vi "INI.Attributes to Variant.vi"(8 "error in (no error)":errorcluster, 9 "Section Attribute":variant, 10 "Data Name":string, 11 "Datatype":variant) -> (0 "error out":errorcluster, 3 "Variant":variant)   [LabVIEW 2013, in "OpenSerializer.lvlib" / "Serializer.PlainText.INI.lvclass"]
doc: "JKI SMO Configuration 1.2.1.18\nJKI - JKI\nCopyright (c) 2017, JKI"
uses:
  Serializer.PlainText.INI.lvclass
  <vilib>/LabVIEW Open Source Project/Data Manipulation/TypeDescriptor/TypeDescriptor_GetName.vi
  <vilib>/LabVIEW Open Source Project/Data Manipulation/Variant/Variant_EmptyCluster.vi
  <vilib>/LabVIEW Open Source Project/Data Manipulation/TypeDescriptor/TypeDescriptor_GetPString.vi
  <vilib>/LabVIEW Open Source Project/Data Manipulation/TypeDescriptor/TypeDescriptor_SetName.vi
  <vilib>/Utility/GetType.llb/TD_Create Cluster.vi
  <vilib>/Utility/GetType.llb/TD_Get Array Information.vi
  <vilib>/Utility/GetType.llb/Get Type Code from I16 Array And Pos.vi
  <vilib>/LabVIEW Open Source Project/Data Manipulation/Conversions/Flattened nD-Array to Flattened 1D-Array.vi
  <vilib>/regexp/Match Regular Expression.xnode
  <vilib>/Utility/VariantDataType/VariantType.lvlib
  <vilib>/LabVIEW Open Source Project/Data Manipulation/Variant/OpenVariant.lvlib
  Serializer.PlainText/Serializer.PlainText.lvclass
  <vilib>/LabVIEW Open Source Project/Data Manipulation/TypeDescriptor/OpenDescriptor.lvlib
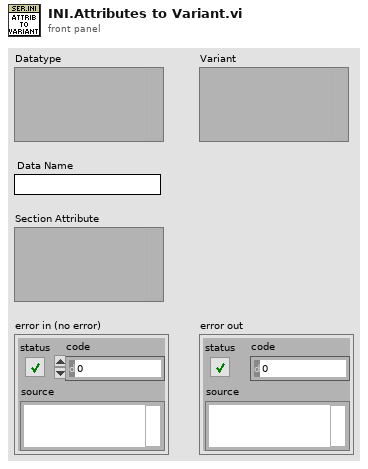
[diagram p1: front panel]
types:
  T1 = typedef "VariantType.lvlib/Type.ctl" = enum8{"Invalid Type", "Void", "I8", "I16", "I32", "I64", "U8", "U16", "U32", "U64", "Single Float", "Double Float", "Extended Float", "Single Complex", "Double Complex", "Extended Complex", "Enum U8", "Enum U16", "Enum U32", "Enum U64", "Single Float With Unit", "Double Float With Unit", "Extended Float With Unit", "Single Complex with Unit", "Double Complex with Unit", "Extended Complex with Unit", "Boolean", "String", "Path", "Picture", "Tag", "Array", "Cluster", "Variant", "LV Variant", "Waveform", "Timestamp", "Digital Waveform", "Digital Data", "ExpressData", "Refnum", "External Data", "VI", "Poly VI", "LabVIEW Class Instance", "Fixed Point"}
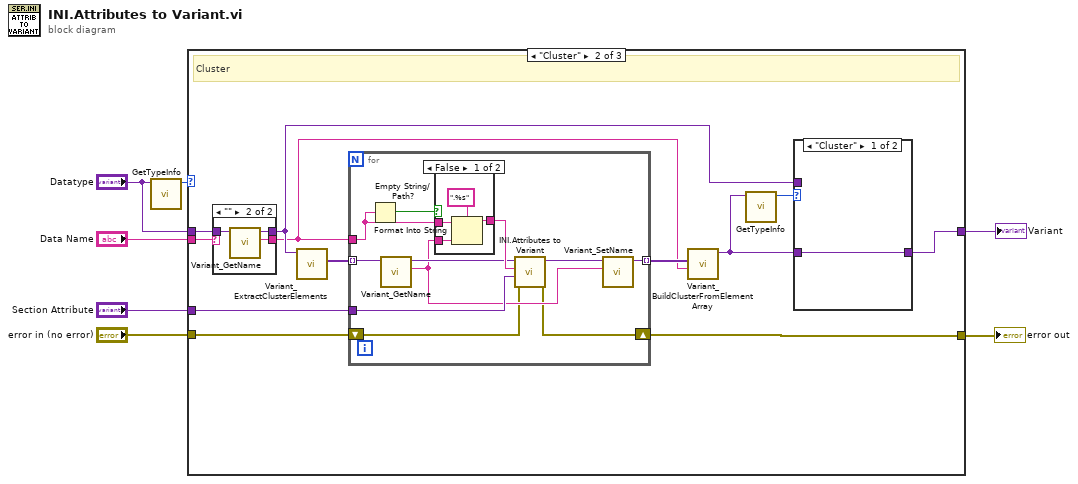
[diagram p0: block diagram]
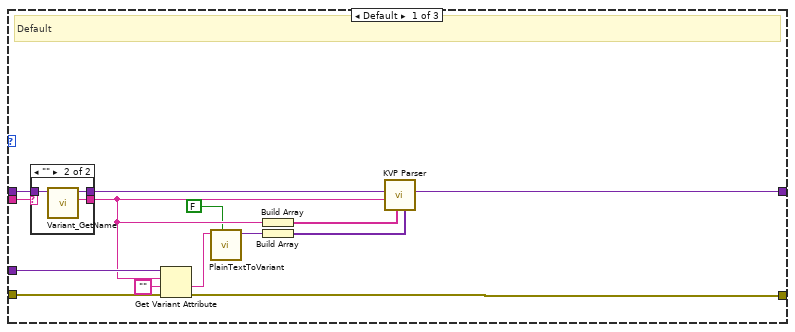
[diagram p2: hidden frame]
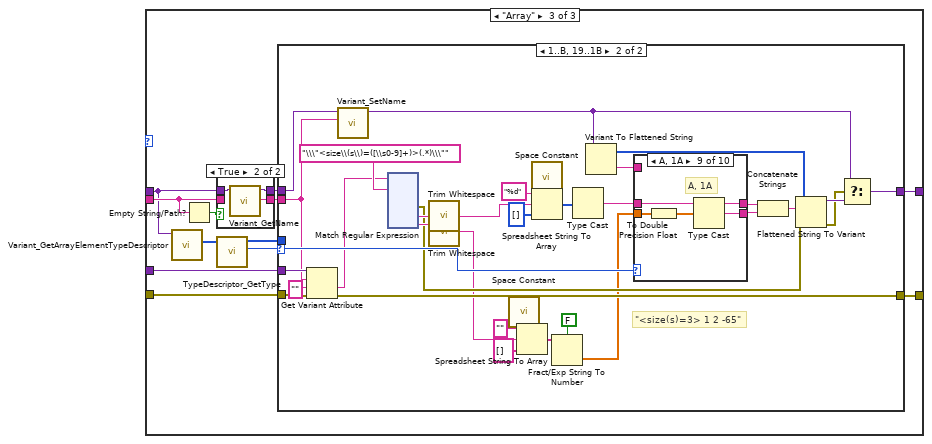
[diagram p7: hidden frame]
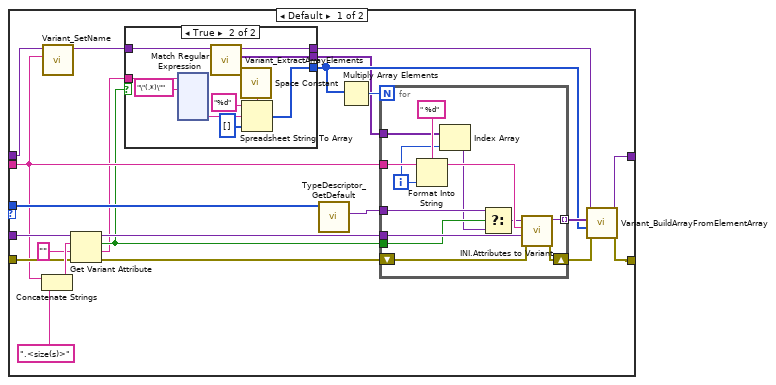
[diagram p9: hidden frame]
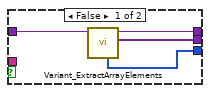
[diagram p10: hidden frame]
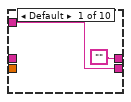
[diagram p11: hidden frame]
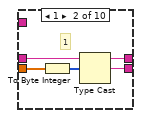
[diagram p12: hidden frame]
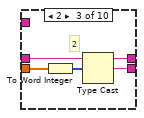
[diagram p13: hidden frame]
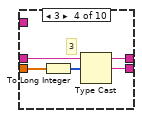
[diagram p14: hidden frame]
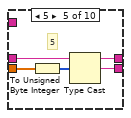
[diagram p15: hidden frame]
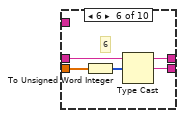
[diagram p16: hidden frame]
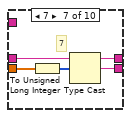
[diagram p17: hidden frame]
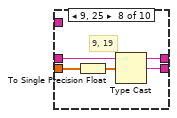
[diagram p18: hidden frame]
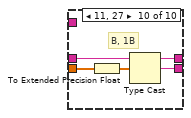
[diagram p19: hidden frame]
diagram:
  n1 = call <vilib>:"GetTypeInfo.vi"("Variant"="Datatype") -> ("Type Enum"=w1:T1)  [unwired: 6 in, 4 out]
  n2 = case shown="\"Cluster\"" w1 {
    tunnel: [w9 w37 w72] -> w3
    tunnel: [w20 w33 w71] -> w4
    tunnel: "Data Name" -> [w18 w27 w67]
    tunnel: "Datatype" -> [w19 w30 w65]
    tunnel: "Section Attribute" -> [w21 w38 w73]
    tunnel: "error in (no error)" -> [w12 w31 w66]
    frame Default {
      # "Default"
      n3 = case shown="\"\"" w18 {
        selector: w18 -> [w22 _]
        tunnel: w19 -> [w23 w25]
        tunnel: [w23 w24] -> w14
        tunnel: [w22 w26] -> w10
        frame Default {
        }
        frame "" {
          n4 = call <vilib>:"Variant_GetName.vi"("Variant"=w25) -> ("Name"=w26:string, "Variant dup"=w24:variant)  [unwired: 8 in, 1 out]
        }
      }
      n5 = Get Variant Attribute(Variant=w21, name=w10, default value (empty Variant)="", error in=w12) -> (value=w11:string, error out=w20:errorcluster)  [unwired: 2 out]
      n6 = call "PlainTextToVariant.vi"("use system decimal point (T)"=FALSE, "String-formatted Value"=w11) -> ("Variant-formatted Value"=w15:variant)  [unwired: 8 in, 1 out]
      n7 = Build Array(w10) -> (w16:string[])
      n8 = Build Array(w15) -> (w17:variant[])
      n9 = call <vilib>:"KVP Parser.vi"("Values"=w17, "Keys"=w16, "Default Value Name (empty: label)"=w10, "Default Value"=w14) -> ("Value"=w9:variant)  [unwired: 4 in, 3 out]
    }
    frame "Cluster" {
      # "Cluster"
      n10 = case shown="\"\"" w27 {
        selector: w27 -> [w39 _]
        tunnel: w30 -> [w40 w42]
        tunnel: [w40 w41] -> w29
        tunnel: [w39 w43] -> w28
        frame Default {
        }
        frame "" {
          n11 = call <vilib>:"Variant_GetName.vi"("Variant"=w42) -> ("Name"=w43:string, "Variant dup"=w41:variant)  [unwired: 8 in, 1 out]
        }
      }
      n12 = call <vilib>:"Variant_ExtractClusterElements.vi"("Cluster"=w29) -> ("Elements"=w32:variant[])  [unwired: 8 in, 2 out]
      n13 = for {
        tunnel: w32 -> [w50] mode=indexing
        shift-right: [w46] -> w33
        shift-left: w31 -> [w47]
        tunnel: w28 -> [w54]
        tunnel: [w51] -> w35 mode=indexing
        tunnel: w38 -> [w55]
        n14 = Empty String/Path?(string/path=w54) -> (empty?=w53:bool)
        n15 = call <vilib>:"Variant_GetName.vi"("Variant"=w50) -> ("Name"=w48:string, "Variant dup"=w49:variant)  [unwired: 8 in, 1 out]
        n16 = case shown="False" w53 {
          tunnel: w48 -> [w59 w61]
          tunnel: [w58 w61] -> w56
          tunnel: w54 -> [w57 _]
          frame False {
            n17 = Format Into String(format string=".%s" ("Format String"), initial string=w57, w59) -> (resulting string=w58:string)  [unwired: 1 in, 1 out]
          }
          frame True {
          }
        }
        n18 = call "INI.Attributes to Variant.vi"("error in (no error)"=w47, "Section Attribute"=w55, "Data Name"=w56, "Datatype"=w49) -> ("error out"=w46:errorcluster, "Variant"=w52:variant)  [unwired: 6 in]
        n19 = call <vilib>:"Variant_SetName.vi"("Name"=w48, "Variant"=w52) -> ("Named Variant"=w51:variant)  [unwired: 9 in]
      }
      n20 = call <vilib>:"Variant_BuildClusterFromElementArray.vi"("name"=w28, "Elements"=w35) -> ("Cluster"=w34:variant)  [unwired: 9 in]
      n21 = call <vilib>:"GetTypeInfo.vi"("Variant"=w34) -> ("Type Enum"=w36:T1)  [unwired: 6 in, 4 out]
      n22 = case shown="\"Cluster\"" w36 {
        tunnel: w29 -> [_ w45]
        tunnel: [w44 w45] -> w37
        tunnel: w34 -> [w44 _]
        frame "Cluster" {
        }
        frame Default {
        }
      }
    }
    frame "Array" {
      n23 = call <vilib>:"Variant_GetArrayElementTypeDescriptor.vi"("Array"=w65) -> ("Element Descriptor"=w64:i16[])  [unwired: 8 in, 2 out]
      n24 = Empty String/Path?(string/path=w67) -> (empty?=w70:bool)
      n25 = case shown="True" w70 {
        tunnel: w65 -> [w74 w78]
        tunnel: [w74 w77] -> w69
        tunnel: [w75 w76] -> w68
        tunnel: w67 -> [w75 _]
        frame False {
        }
        frame True {
          n26 = call <vilib>:"Variant_GetName.vi"("Variant"=w78) -> ("Name"=w76:string, "Variant dup"=w77:variant)  [unwired: 8 in, 1 out]
        }
      }
      n27 = call <vilib>:"TypeDescriptor_GetType.vi"("type descriptor"=w64) -> ("Type"=w62:u8, "type descriptor dup"=w63:i16[])  [unwired: 9 in]
      n28 = case shown="1..B, 19..1B" w62 {
        selector: w62 -> [_ w265]
        tunnel: w69 -> [w82 w251]
        tunnel: [w89 w266] -> w72
        tunnel: [w87 w255] -> w71
        tunnel: w73 -> [w98 w276]
        tunnel: w66 -> [w92 w274]
        tunnel: w68 -> [w86 w252]
        tunnel: w63 -> [w91 _]
        frame Default {
          n29 = Concatenate Strings(w86, ".<size(s)>" ("Substring")) -> (w97:string)
          n30 = call <vilib>:"Variant_SetName.vi"("Name"=w86, "Variant"=w82) -> ("Named Variant"=w80:variant)  [unwired: 9 in]
          n31 = Get Variant Attribute(Variant=w98, name=w97, default value (empty Variant)="" ("Substring")) -> (duplicate Variant=w94:variant, found=w85:bool, value=w84:string)  [unwired: 1 in, 1 out]
          n32 = case shown="True" w85 {
            tunnel: w84 -> [_ w112]
            tunnel: [w100 w107] -> w83
            tunnel: w80 -> [w103 w106]
            tunnel: [w102 w105] -> w81
            tunnel: [w101 w104] -> w79
            frame False {
              n33 = call <vilib>:"Variant_ExtractArrayElements.vi"("Array"=w103) -> ("Elements"=w102:variant[], "Array dup"=w101:variant, "Dimensions"=w100:u32[])  [unwired: 7 in, 1 out]
            }
            frame True {
              n34 = xnode "Match Regular Expression"("input string"=w112, "regular expression"="\"(.*)\"") -> ("submatch 1"=w108:string)  [unwired: 4 in, 5 out]
              n35 = call <vilib>:"Variant_ExtractArrayElements.vi"("Array"=w106) -> ("Elements"=w105:variant[], "Array dup"=w104:variant)  [unwired: 7 in, 2 out]
              n36 = call <vilib>:"Space Constant.vi"() -> ("String"=w111:string)
              n37 = Spreadsheet String To Array(delimiter (Tab)=w111, format string="%d", spreadsheet string=w108, array type (2D Dbl)=u32[] [] ("Array Constant")) -> (array=w107:u32[])
            }
          }
          n38 = call <vilib>:"TypeDescriptor_GetDefault.vi"("type descriptor"=w91) -> ("Default"=w93:variant)  [unwired: 8 in, 2 out]
          n39 = Multiply Array Elements(1:w83) -> (0:w95:u32)
          n40 = for {
            N: w95 -> [_]
            tunnel: w94 -> [w242]
            tunnel: w93 -> [w234]
            tunnel: [w241] -> w90 mode=indexing
            tunnel: w86 -> [w238]
            shift-right: [w230] -> w88
            shift-left: w92 -> [w231]
            tunnel: w81 -> [w237]
            tunnel: w85 -> [w235]
            i -> [w236]
            n41 = Format Into String(format string=" %d" ("Format String"), initial string=w238, w236) -> (resulting string=w239:string)  [unwired: 1 in, 1 out]
            n42 = Index Array(array=w237, index=w236) -> (element=w233:variant)
            n43 = Select(t=w234, s=w235, f=w233) -> (s? t:f=w232:variant)
            n44 = call "INI.Attributes to Variant.vi"("error in (no error)"=w231, "Section Attribute"=w242, "Data Name"=w239, "Datatype"=w232) -> ("error out"=w230:errorcluster, "Variant"=w241:variant)  [unwired: 6 in]
          }
          n45 = call <vilib>:"Variant_BuildArrayFromElementArray.vi"("error in (no error)"=w88, "Dimensions"=w83, "Elements"=w90, "Default Array"=w79) -> ("error out"=w87:errorcluster, "Output Array"=w89:variant)  [unwired: 6 in]
        }
        frame 1..11, 25..27 {
          # "\"<size(s)=3> 1 2 -65\""
          n46 = Get Variant Attribute(Variant=w276, name=w252, default value (empty Variant)="", error in=w274) -> (value=w258:string, error out=w255:errorcluster)  [unwired: 2 out]
          n47 = call <vilib>:"Variant_SetName.vi"("Name"=w252, "Variant"=w251) -> ("Named Variant"=w250:variant)  [unwired: 9 in]
          n48 = xnode "Match Regular Expression"("input string"=w258, "regular expression"="\\\"<size\\(s\\)=([\\s0-9]+)>(.*)\\\"") -> ("error out"=w253:errorcluster, "submatch 1"=w260:string, "submatch 2"=w261:string)  [unwired: 4 in, 4 out]
          n49 = call <vilib>:"Trim Whitespace.vi"("string"=w260) -> ("trimmed string"=w257:string)  [unwired: 1 in]
          n50 = call <vilib>:"Trim Whitespace.vi"("string"=w261) -> ("trimmed string"=w244:string)  [unwired: 1 in]
          n51 = call <vilib>:"Space Constant.vi"() -> ("String"=w247:string)
          n52 = Spreadsheet String To Array(delimiter (Tab)=w247, format string="", spreadsheet string=w244, array type (2D Dbl)=string[] []) -> (array=w246:string[])
          n53 = call <vilib>:"Space Constant.vi"() -> ("String"=w254:string)
          n54 = Spreadsheet String To Array(delimiter (Tab)=w254, format string="%d", spreadsheet string=w257, array type (2D Dbl)=u32[] []) -> (array=w264:u32[])
          n55 = Fract/Exp String To Number(use system decimal point (T)=FALSE, string=w246) -> (number=w243:dbl[])  [unwired: 2 in, 1 out]
          n56 = Type Cast(x=w264) -> (*(type *) &x=w256:string)  [unwired: 1 in]
          n57 = Variant To Flattened String(Variant=w250) -> (data string=w271:string, 1:w270:i16[])
          n58 = case shown="A, 1A" w265 {
            tunnel: w243 -> [_ w399 w403 w407 w411 w415 w419 w423 w425 w429]
            tunnel: [w394 w397 w401 w405 w409 w413 w417 w421 w427 w431] -> w268
            tunnel: ["" w396 w400 w404 w408 w412 w416 w420 w426 w430] -> w269
            tunnel: w256 -> [_ w396 w400 w404 w408 w412 w416 w420 w426 w430]
            tunnel: w271 -> [w394 _ _ _ _ _ _ _ _ _]
            frame Default {
            }
            frame 1 {
              # "1"
              n59 = To Byte Integer(number=w399) -> (8bit integer=w398:i8[])
              n60 = Type Cast(x=w398) -> (*(type *) &x=w397:string)  [unwired: 1 in]
            }
            frame 2 {
              # "2"
              n61 = To Word Integer(number=w403) -> (16bit integer=w402:i16[])
              n62 = Type Cast(x=w402) -> (*(type *) &x=w401:string)  [unwired: 1 in]
            }
            frame 3 {
              # "3"
              n63 = To Long Integer(number=w407) -> (32bit integer=w406:i32[])
              n64 = Type Cast(x=w406) -> (*(type *) &x=w405:string)  [unwired: 1 in]
            }
            frame 5 {
              # "5"
              n65 = To Unsigned Byte Integer(number=w411) -> (unsigned 8bit integer=w410:u8[])
              n66 = Type Cast(x=w410) -> (*(type *) &x=w409:string)  [unwired: 1 in]
            }
            frame 6 {
              # "6"
              n67 = To Unsigned Word Integer(number=w415) -> (unsigned 16bit integer=w414:u16[])
              n68 = Type Cast(x=w414) -> (*(type *) &x=w413:string)  [unwired: 1 in]
            }
            frame 7 {
              # "7"
              n69 = To Unsigned Long Integer(number=w419) -> (unsigned 32bit integer=w418:u32[])
              n70 = Type Cast(x=w418) -> (*(type *) &x=w417:string)  [unwired: 1 in]
            }
            frame 9, 25 {
              # "9, 19"
              n71 = To Single Precision Float(number=w423) -> (single precision float=w422:sgl[])
              n72 = Type Cast(x=w422) -> (*(type *) &x=w421:string)  [unwired: 1 in]
            }
            frame 10, 26 {
              # "A, 1A"
              n73 = To Double Precision Float(number=w425) -> (double precision float=w424:dbl[])
              n74 = Type Cast(x=w424) -> (*(type *) &x=w427:string)  [unwired: 1 in]
            }
            frame 11, 27 {
              # "B, 1B"
              n75 = To Extended Precision Float(1:w429) -> (0:w428:ext[])
              n76 = Type Cast(x=w428) -> (*(type *) &x=w431:string)  [unwired: 1 in]
            }
          }
          n77 = Concatenate Strings(w269, w268) -> (w267:string)
          n78 = Flattened String To Variant(4:w253, 6:w267, 7:w270) -> (0:w272:errorcluster, 3:w273:variant)
          n79 = Select(t=w250, s=w272, f=w273) -> (s? t:f=w266:variant)
        }
      }
    }
  }
  "error out" <- w4
  "Variant" <- w3
